vi "objTrackerMasksub.vi"(4 "B Color":i16, 6 "G Color":i16, 8 "R Color":i16, 10 "Mask In":T1 {"Dialogs" format="%.0b"}, 11 "Original Image":T1 {"Dialogs" format="%.0b"}) -> (3 "image Out":picture)   [LabVIEW 2012]
uses:
  <userlib>/ImageProcessing/QTLIB_2595_LV86/QT_Image.ctl
  <userlib>/ImageProcessing/LV86_MaskImage.vi
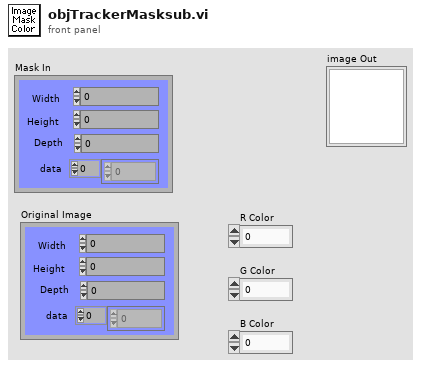
[diagram p1: front panel]
types:
  T1 = typedef "QT_Image.ctl" = cluster{"Width":i32, "Height":i32, "Depth":i32, "data":u8[], "Compressed data":u8[], "Color table":u32[], "Duration":i32, "Options":i32, "Timestamp":i32, "ID":i32, "Reserved":i32, "Dialogs":u32}
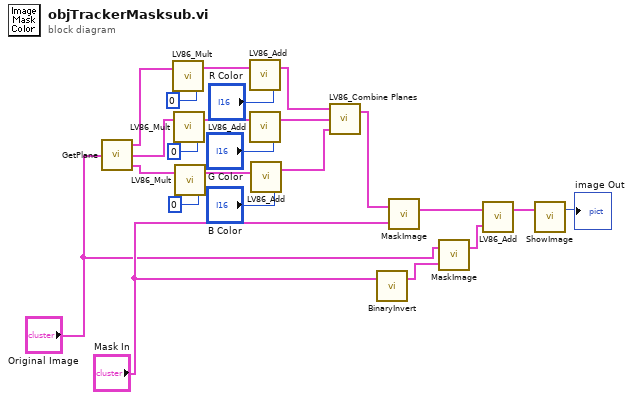
[diagram p0: block diagram]
diagram:
  n1 = call <userlib>:"GetPlane.vi"("Image In"="Original Image") -> ("Blue Plane Out"=w7:T1, "Green Plane Out"=w6:T1, "Red Plane Out"=w2:T1)
  n2 = call <userlib>:"LV86_Mult.vi"("Constant"=i16 0, "Image"=w2) -> ("Image Out"=w8:T1)  [unwired: 1 in]
  n3 = call <userlib>:"LV86_Mult.vi"("Constant"=i16 0, "Image"=w6) -> ("Image Out"=w11:T1)  [unwired: 1 in]
  n4 = call <userlib>:"LV86_Mult.vi"("Constant"=i16 0, "Image"=w7) -> ("Image Out"=w13:T1)  [unwired: 1 in]
  n5 = call <userlib>:"LV86_Add.vi"("Constant"="R Color", "Image"=w8) -> ("Image Out"=w14:T1)  [unwired: 1 in]
  n6 = call <userlib>:"LV86_Add.vi"("Constant"="G Color", "Image"=w11) -> ("Image Out"=w15:T1)  [unwired: 1 in]
  n7 = call <userlib>:"LV86_Add.vi"("Constant"="B Color", "Image"=w13) -> ("Image Out"=w16:T1)  [unwired: 1 in]
  n8 = call <userlib>:"LV86_Combine Planes.vi"("Blue"=w16, "Green"=w15, "Red"=w14) -> ("Image 2"=w17:T1)  [unwired: 1 in]
  n9 = call <userlib>:"BinaryInvert.vi"("Image In"="Mask In") -> ("Image Out"=w22:T1)  [unwired: 2 in]
  n10 = call-poly <userlib>:"MaskImage.vi"("Mask in"="Mask In", "Image"=w17) -> ("Image Out"=w19:T1)  [unwired: 1 in]
  n11 = call-poly <userlib>:"MaskImage.vi"("Mask in"=w22, "Image"="Original Image") -> ("Image Out"=w20:T1)  [unwired: 1 in]
  n12 = call <userlib>:"LV86_Add.vi"("Image 2"=w20, "Image"=w19) -> ("Image Out"=w18:T1)  [unwired: 1 in]
  n13 = call <userlib>:"ShowImage.vi"("Image"=w18) -> ("image"=→"image Out":picture)  [unwired: 2 in, 1 out]
